vi "duplicateNodes.vi"(8 "error in (no error)":errorcluster, 10 "Node Path":string, 11 "xceRootNode in":refnum<class "xceRootNode.lvclass">) -> (0 "error out":errorcluster, 3 "xceRootNode out":refnum<class "xceRootNode.lvclass">)   [LabVIEW 2013, in "xceRootNode.lvclass"]
doc: "Duplicates a node in the tree data structure, and the tree control."
uses:
  xceRootNode.lvclass
  xceNode/xceNode.lvclass
  xceDataNode/xceDataNode.lvclass
  xceRootNode.lvclass/xceRootNode.ctl
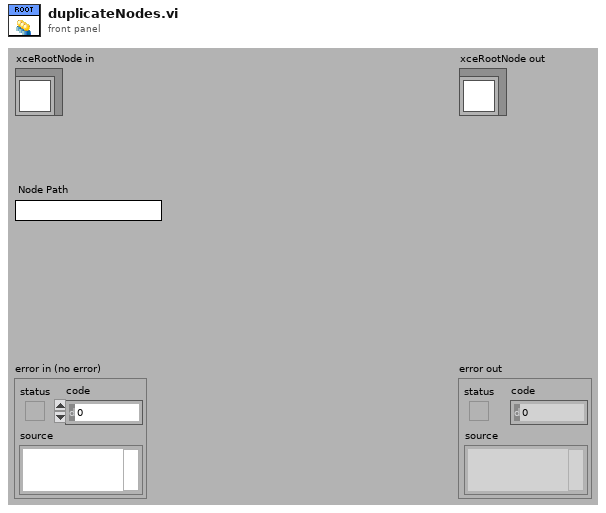
[diagram p1: front panel]
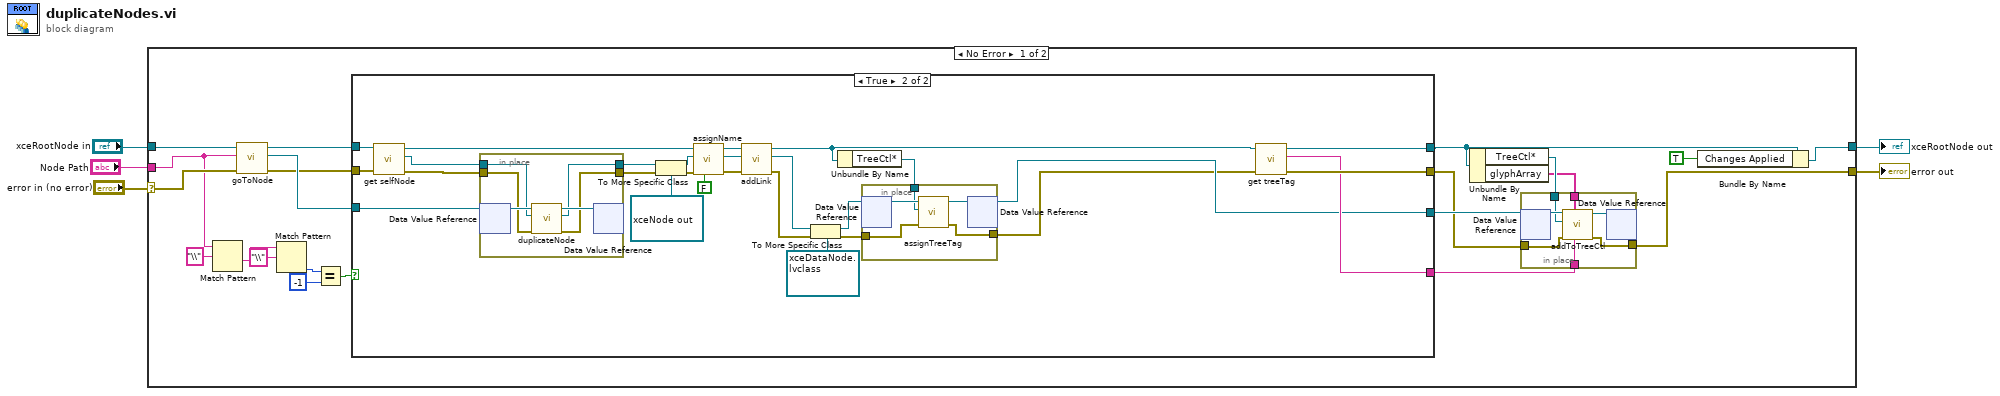
[diagram p0: block diagram]
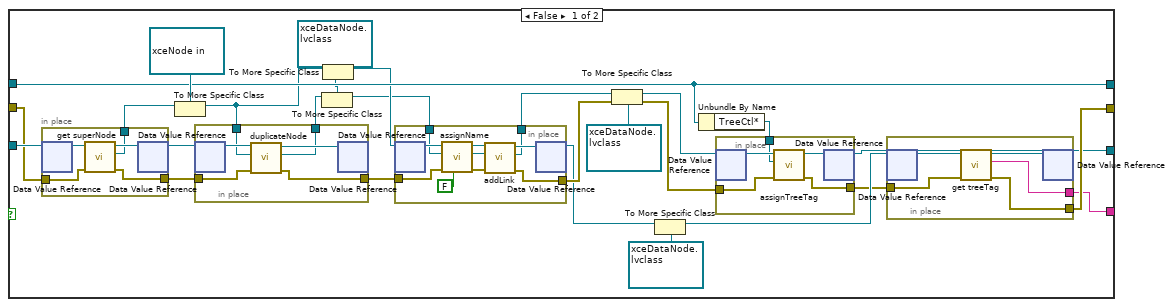
[diagram p2: hidden frame]
diagram:
  n1 = case shown="No Error" "error in (no error)" {
    selector: "error in (no error)" -> [w25 w130]
    tunnel: [w12 w130] -> w4
    tunnel: [w7 w129] -> w2
    tunnel: "xceRootNode in" -> [w26 w129]
    tunnel: "Node Path" -> [w23 _]
    frame No Error {
      n2 = Match Pattern(string=w23, regular expression="\\") -> (after substring=w21:string)  [unwired: 1 in, 3 out]
      n3 = call "goToNode.vi"("error in (no error)"=w25, "Node Path"=w23, "xceNode in"=w26) -> ("error out"=w15:errorcluster, "goToNode* out"=w24:refnum<data-value>, "xceNode out"=w16:refnum<class "xceRootNode.lvclass">)  [unwired: 6 in]
      n4 = Match Pattern(string=w21, regular expression="\\") -> (offset past match=w19:i32)  [unwired: 1 in, 3 out]
      n5 = Equal?(x=w19, y=-1) -> (x = y?=w17:bool)
      n6 = case shown="True" w17 {
        tunnel: w24 -> [w52 w110]
        tunnel: w16 -> [w41 w109]
        tunnel: w15 -> [w51 w108]
        tunnel: [w41 w99] -> w9
        tunnel: [w34 w98] -> w13
        tunnel: [w27 w96] -> w14
        tunnel: [w33 w97] -> w10
        frame False {
          w30 = refnum<data-value> refnum ("data value reference")
          n7 = in-place {
            in-place-border: w51 -> [w82]
            in-place-border: [w80] -> w49
            in-place-border: [w79] -> w47
            n8 = in-place-dvr #1(w52) -> (w83:refnum<class "xceNode.lvclass">)  [unwired: 1 out]
            n9 = call "get superNode.vi"("error in (no error)"=w82, "xceNode in"=w83) -> ("error out"=w79:errorcluster, "superNode*"=w80:refnum<data-value>, "xceNode out"=w81:refnum<class "xceNode.lvclass">)  [unwired: 7 in]
            n10 = in-place-dvr #1(w81) -> (w50:refnum<data-value>)  [unwired: 1 out]
          }
          n11 = To More Specific Class(target class=refnum<data-value> refnum ("goToNode* out"), reference=w49) -> (specific class reference=w31:refnum<data-value>)  [unwired: 1 in, 1 out]
          n12 = in-place {
            in-place-border: w31 -> [w76]
            in-place-border: [w75] -> w29
            in-place-border: w47 -> [w74]
            in-place-border: [w73] -> w46
            n13 = in-place-dvr #2(w50) -> (w78:refnum<class "xceNode.lvclass">)  [unwired: 1 out]
            n14 = call "duplicateNode.vi"("error in (no error)"=w74, "superNode*"=w76, "xceNode in"=w78) -> ("error out"=w73:errorcluster, "duplicateNode*"=w75:refnum<data-value>, "xceNode out"=w77:refnum<class "xceNode.lvclass">)  [unwired: 6 in]
            n15 = in-place-dvr #2(w77) -> ()  [unwired: 2 out]
          }
          n16 = To More Specific Class(target class=w30, reference=w29) -> (specific class reference=w28:refnum<data-value>)  [unwired: 1 in, 1 out]
          n17 = To More Specific Class(target class=w30, reference=w31) -> (specific class reference=w32:refnum<data-value>)  [unwired: 1 in, 1 out]
          n18 = in-place {
            in-place-border: w28 -> [w65]
            in-place-border: w46 -> [w67]
            in-place-border: [w71] -> w43
            in-place-border: [w70] -> w44
            n19 = in-place-dvr #3(w32) -> (w69:refnum<class "xceDataNode.lvclass">)  [unwired: 1 out]
            n20 = call "assignName.vi"("recurse"=FALSE, "error in (no error)"=w67, "subNode in"=w65, "superNode in"=w69) -> ("error out"=w66:errorcluster, "subNode out"=w64:refnum<data-value>, "superNode out"=w68:refnum<class "xceDataNode.lvclass">)  [unwired: 5 in]
            n21 = call "addLink.vi"("error in (no error)"=w66, "subNode in"=w64, "superNode in"=w68) -> ("error out"=w71:errorcluster, "subNode out"=w70:refnum<data-value>, "superNode out"=w72:refnum<class "xceDataNode.lvclass">)  [unwired: 6 in]
            n22 = in-place-dvr #3(w72) -> (w37:refnum<data-value>)  [unwired: 1 out]
          }
          n23 = To More Specific Class(target class=refnum<data-value> refnum ("data value reference"), reference=w44, error in=w43) -> (specific class reference=w40:refnum<data-value>, error out=w39:errorcluster)
          n24 = To More Specific Class(target class=refnum<data-value> refnum ("data value reference"), reference=w37) -> (specific class reference=w36:refnum<data-value>)  [unwired: 1 in, 1 out]
          n25 = Unbundle By Name(w41) -> ("TreeCtl*"=w42:refnum<vi>)
          n26 = in-place {
            in-place-border: w39 -> [w61]
            in-place-border: w42 -> [w59]
            in-place-border: [w58] -> w35
            n27 = in-place-dvr #4(w40) -> (w62:refnum<class "xceDataNode.lvclass">)  [unwired: 1 out]
            n28 = call "assignTreeTag.vi"("error in (no error)"=w61, "TreeCtl*"=w59, "xceDataNode in"=w62) -> ("error out"=w58:errorcluster, "xceDataNode out"=w60:refnum<class "xceDataNode.lvclass">)  [unwired: 7 in]
            n29 = in-place-dvr #4(w60) -> (w27:refnum<data-value>)  [unwired: 1 out]
          }
          n30 = in-place {
            in-place-border: w35 -> [w53]
            in-place-border: [w56] -> w34
            in-place-border: [w55] -> w33
            n31 = in-place-dvr #5(w36) -> (w54:refnum<class "xceDataNode.lvclass">)  [unwired: 1 out]
            n32 = call "get treeTag.vi"("error in (no error)"=w53, "xceNode in"=w54) -> ("error out"=w56:errorcluster, "treeTag"=w55:string, "xceNode out"=w57:refnum<class "xceDataNode.lvclass">)  [unwired: 7 in]
            n33 = in-place-dvr #5(w57) -> ()  [unwired: 2 out]
          }
        }
        frame True {
          n34 = call "get selfNode.vi"("error in (no error)"=w108, "xceNode in"=w109) -> ("error out"=w100:errorcluster, "selfNode*"=w101:refnum<data-value>, "xceNode out"=w89:refnum<class "xceRootNode.lvclass">)  [unwired: 7 in]
          n35 = in-place {
            in-place-border: [w119] -> w92
            in-place-border: w101 -> [w117]
            in-place-border: w100 -> [w118]
            in-place-border: [w116] -> w86
            n36 = in-place-dvr #6(w110) -> (w121:refnum<class "xceNode.lvclass">)  [unwired: 1 out]
            n37 = call "duplicateNode.vi"("error in (no error)"=w118, "superNode*"=w117, "xceNode in"=w121) -> ("error out"=w116:errorcluster, "duplicateNode*"=w119:refnum<data-value>, "xceNode out"=w120:refnum<class "xceNode.lvclass">)  [unwired: 6 in]
            n38 = in-place-dvr #6(w120) -> ()  [unwired: 2 out]
          }
          n39 = To More Specific Class(target class=refnum<data-value> refnum ("subNode in"), reference=w92, error in=w86) -> (specific class reference=w90:refnum<data-value>, error out=w85:errorcluster)
          n40 = call "assignName.vi"("recurse"=FALSE, "error in (no error)"=w85, "subNode in"=w90, "superNode in"=w89) -> ("error out"=w93:errorcluster, "subNode out"=w87:refnum<data-value>, "superNode out"=w88:refnum<class "xceRootNode.lvclass">)  [unwired: 5 in]
          n41 = call "addLink.vi"("error in (no error)"=w93, "subNode in"=w87, "superNode in"=w88) -> ("error out"=w103:errorcluster, "subNode out"=w105:refnum<data-value>, "superNode out"=w94:refnum<class "xceRootNode.lvclass">)  [unwired: 6 in]
          n42 = To More Specific Class(target class=refnum<data-value> refnum ("data value reference"), reference=w105, error in=w103) -> (specific class reference=w104:refnum<data-value>, error out=w102:errorcluster)
          n43 = Unbundle By Name(w94) -> ("TreeCtl*"=w107:refnum<vi>)
          n44 = in-place {
            in-place-border: w102 -> [w114]
            in-place-border: w107 -> [w112]
            in-place-border: [w111] -> w95
            n45 = in-place-dvr #7(w104) -> (w115:refnum<class "xceDataNode.lvclass">)  [unwired: 1 out]
            n46 = call "assignTreeTag.vi"("error in (no error)"=w114, "TreeCtl*"=w112, "xceDataNode in"=w115) -> ("error out"=w111:errorcluster, "xceDataNode out"=w113:refnum<class "xceDataNode.lvclass">)  [unwired: 7 in]
            n47 = in-place-dvr #7(w113) -> (w96:refnum<data-value>)  [unwired: 1 out]
          }
          n48 = call "get treeTag.vi"("error in (no error)"=w95, "xceNode in"=w94) -> ("error out"=w98:errorcluster, "treeTag"=w97:string, "xceNode out"=w99:refnum<class "xceRootNode.lvclass">)  [unwired: 7 in]
        }
      }
      n49 = Unbundle By Name(w9) -> ("TreeCtl*"=w11:refnum<vi>, "glyphArray"=w6:string[])
      n50 = in-place {
        in-place-border: w13 -> [w126]
        in-place-border: [w125] -> w12
        in-place-border: w11 -> [w124]
        in-place-border: w10 -> [w123]
        in-place-border: w6 -> [w122]
        n51 = in-place-dvr #8(w14) -> (w127:refnum<class "xceDataNode.lvclass">)  [unwired: 1 out]
        n52 = call "addToTreeCtl.vi"("ParentTreeTag"=w123, "glyphArray"=w122, "error in (no error)"=w126, "TreeCtl*"=w124, "xceDataNode in"=w127) -> ("error out"=w125:errorcluster, "xceDataNode out"=w128:refnum<class "xceDataNode.lvclass">)  [unwired: 5 in]
        n53 = in-place-dvr #8(w128) -> ()  [unwired: 2 out]
      }
      n54 = Bundle By Name(cluster=w9, "Changes Applied"=TRUE) -> (w7:refnum<class "xceRootNode.lvclass">)
    }
    frame Error {
    }
  }
  "error out" <- w4
  "xceRootNode out" <- w2
